vi "Zapis tabeli do pliku.vi"(7 "1d array in":string[](array[string]), 9 "2d array in":string[][](array[string])) -> (1 "for 1d array out":string, 3 "for 2d array out":string)   [LabVIEW 2015]
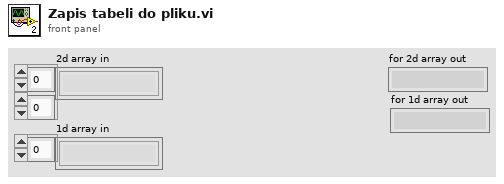
[diagram p1: front panel]
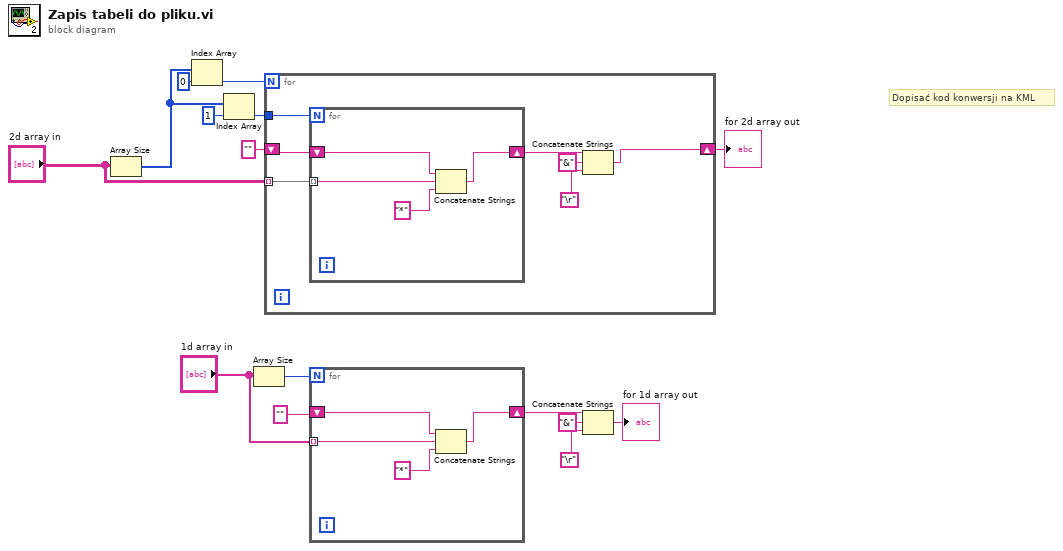
[diagram p0: block diagram]
diagram:
  # "Dopisać kod konwersji na KML"
  n1 = Array Size(array="2d array in") -> (size(s)=w15:i32[])
  n2 = Index Array(array=w15, index=0) -> (element=w11:i32)
  n3 = Index Array(array=w15, index=1) -> (element=w12:i32)
  n4 = Array Size(array="1d array in") -> (size(s)=w4:i32)
  n5 = for {
    N: w11 -> [_]
    tunnel: w12 -> [w22]
    tunnel: "2d array in" -> [w21] mode=indexing
    shift-right: [w17] -> w8
    shift-left: "" -> [w16]
    n6 = for {
      N: w22 -> [_]
      tunnel: w21 -> [w26] mode=indexing
      shift-right: [w24] -> w20
      shift-left: w16 -> [w23]
      n7 = Concatenate Strings(w23, w26, "*") -> (w24:string)
    }
    n8 = Concatenate Strings(w20, "&" ("string"), "\r") -> (w17:string)
  }
  "for 2d array out" <- w8
  n9 = for {
    N: w4 -> [_]
    tunnel: "1d array in" -> [w30] mode=indexing
    shift-right: [w28] -> w5
    shift-left: "" -> [w27]
    n10 = Concatenate Strings(w27, w30, "*") -> (w28:string)
  }
  n11 = Concatenate Strings(w5, "&" ("string"), "\r") -> (→"for 1d array out":string)
